vi "Scale Tags.vi"(11 "Scale Module Configs":T1[](array[typedef])) -> (1 "All Boolean Tags 2":string[](array[string]), 2 "Scale Tags Array":T5(array[cluster]), 3 "All  Numeric Tags 2":string[](array[string]))   [LabVIEW 2018]
uses:
  Scale Module Folder/Feed Module/Controls/Scale Module Config Cluster.ctl
  <vilib>/Utility/miscctls.llb/LVPoint32TypeDef.ctl
  Scale Module Folder/Feed Module/Controls/Scale Module Settings Cluster.ctl
  Mettler Toledo/Controls/Settings Cluster.ctl
  Scale Class/Scale Module Tag Names.ctl
  Scale Module Folder/Scale Module.lvlib
  Mettler Toledo/Mettler Toledo.lvlib
panel:
  # "Scale Settings"
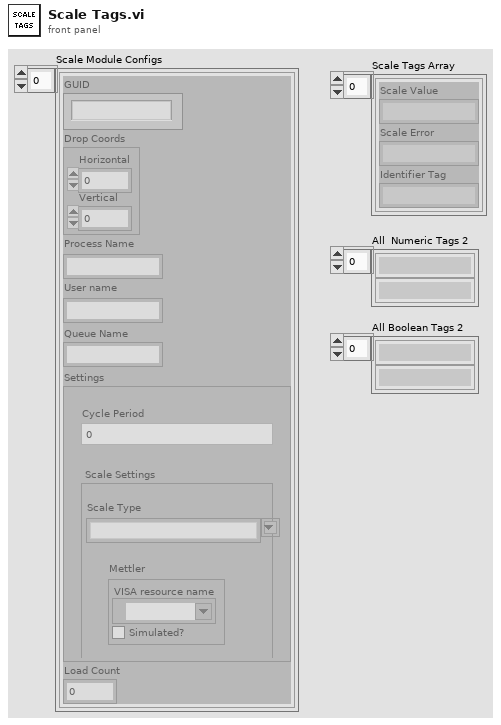
[diagram p1: front panel]
types:
  T1 = typedef "Scale Module.lvlib/Scale Module Config Cluster.ctl" = cluster{"GUID":string, "Drop Coords":T2, "Process Name":string, "User name":string, "Queue Name":string, "Settings":T3, "Load Count":i32}
  T2 = typedef "LVPoint32TypeDef.ctl" = cluster{"Horizontal":i32, "Vertical":i32}
  T3 = typedef "Scale Module.lvlib/Scale Module Settings Cluster.ctl" = cluster{"Cycle Period":dbl, "Mettler":T4, "Scale Type":string}
  T4 = typedef "Mettler Toledo.lvlib/Settings Cluster.ctl" = cluster{"VISA resource name":refnum<visa-resource-name>, "Simulated?":bool}
  T5 = cluster{"Scale Value":string, "Scale Error":string, "Identifier Tag":string}[]
  T6 = typedef "Scale Module.lvlib/Scale Module Tag Names.ctl" = cluster{"Scale Value":string, "Scale Error":string, "Identifier Tag":string}
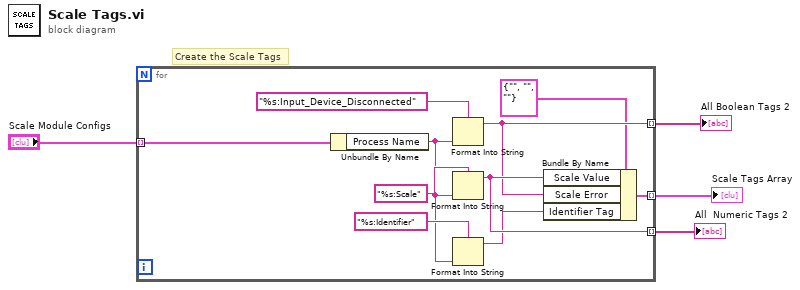
[diagram p0: block diagram]
diagram:
  # "Create the Scale Tags"
  n1 = for {
    tunnel: "Scale Module Configs" -> [w9] mode=indexing
    tunnel: [w10] -> w4 mode=indexing
    tunnel: [w12] -> w2 mode=indexing
    tunnel: [w11] -> w1 mode=indexing
    n2 = Unbundle By Name(w9) -> ("Process Name"=w7:string)
    n3 = Format Into String(format string="%s:Input_Device_Disconnected", w7) -> (resulting string=w11:string)  [unwired: 2 in, 1 out]
    n4 = Format Into String(format string="%s:Scale", w7) -> (resulting string=w12:string)  [unwired: 2 in, 1 out]
    n5 = Format Into String(format string="%s:Identifier", w7) -> (resulting string=w6:string)  [unwired: 2 in, 1 out]
    n6 = Bundle By Name(cluster=T6 {"Scale Value"="", "Scale Error"="", "Identifier Tag"=""} ("Scale Tags 2"), "Scale Value"=w12, "Scale Error"=w11, "Identifier Tag"=w6) -> (w10:T6)
  }
  "Scale Tags Array" <- w4
  "All  Numeric Tags 2" <- w2
  "All Boolean Tags 2" <- w1
